vi "Configure_Interrupt_Duration.vi"(7 "I2C Channel":u8, 8 "error in":errorcluster, 9 "Interrupt Threshold":u8, 10 "Interrupt Source":T1(ring), 11 "LINX Resource In":T2) -> (0 "error out":errorcluster, 2 "ODR-adjusted Duration (s)":dbl, 3 "LINX Resource Out":T2)   [LabVIEW 2014, in "LMH-LINX.lvlib" / "LIS331HH.lvlib"]
uses:
  <vilib>/MakerHub/LINX/Public/Sensors/Accelerometer/LIS331HH/LIS331HH.lvlib
  <vilib>/MakerHub/LINX/Private/Type Defs/LINX Ref.ctl
  <vilib>/MakerHub/LINX/Private/Type Defs/Platform.ctl
  <vilib>/MakerHub/LINX/Private/Type Defs/Interface.ctl
  <vilib>/MakerHub/LINX/Private/Device/Type Defs/LINX Device Config.ctl
  <vilib>/MakerHub/LINX/Private/Device/Type Defs/TCP Config.ctl
  <vilib>/MakerHub/LINX/Private/Device/Type Defs/Channels.ctl
  <vilib>/MakerHub/LINX/Private/Local IO/LinxI2cWrite.vi
  <vilib>/MakerHub/LINX/Public/Utilities/Check Channel.vi
  <vilib>/MakerHub/LINX/Private/Utilties/Generate Error.vi
  <vilib>/MakerHub/LINX/LMH-LINX.lvlib
  <vilib>/MakerHub/LINX/Private/Device/Device.lvlib
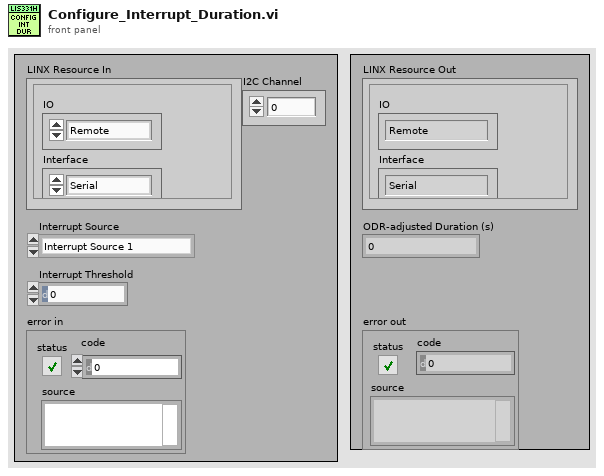
[diagram p1: front panel]
types:
  T1 = enum16{"Interrupt Source 1", "Interrupt Source 2"}
  T2 = typedef "LMH-LINX.lvlib/LINX Ref.ctl" = cluster{"IO":T3, "Interface":T4, "LINX Device Config":T5}
  T3 = typedef "LMH-LINX.lvlib/Platform.ctl" = enum16{"Remote", "Local"}
  T4 = typedef "LMH-LINX.lvlib/Interface.ctl" = enum16{"Serial", "TCP"}
  T5 = typedef "LMH-LINX.lvlib/Device.lvlib/LINX Device Config.ctl" = cluster{"Interface":T4, "COM Port":refnum<visa-resource-name>, "TCP Configuration":T6, "Device Family":u8, "Device ID":u8, "Device Name":string, "TCP Ref":refnum<k5>, "Channels":T7}
  T6 = typedef "LMH-LINX.lvlib/Device.lvlib/TCP Config.ctl" = cluster{"IP Address":string, "Port":u16}
  T7 = typedef "LMH-LINX.lvlib/Channels.ctl" = cluster{"DI":u8[], "DO":u8[], "AI":u8[], "AO":u8[], "PWM":u8[], "QE":u8[], "UART":u8[], "I2C 2":u8[], "SPI":u8[], "CAN":u8[], "Servo":u8[], "AI Ref (V)":dbl, "AI Resolution (Bits)":u8, "AO Ref (V)":dbl, "AO Resolution (Bits)":u8}
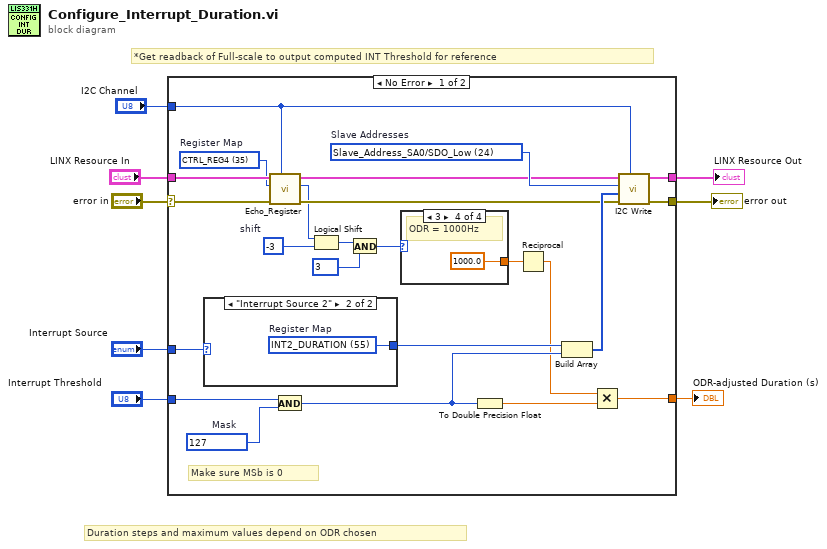
[diagram p0: block diagram]
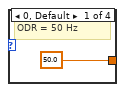
[diagram p2: hidden frame]
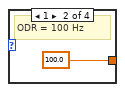
[diagram p3: hidden frame]
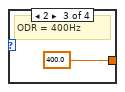
[diagram p4: hidden frame]
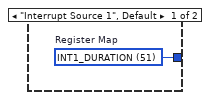
[diagram p5: hidden frame]
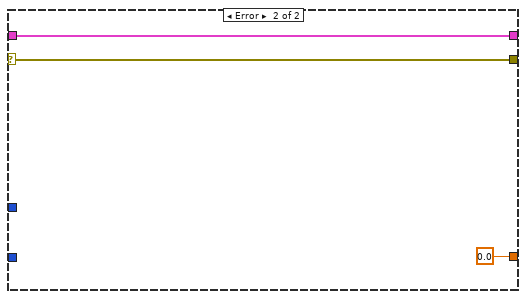
[diagram p6: hidden frame]
diagram:
  # "*Get readback of Full-scale to output computed INT Threshold for reference"
  # "Duration steps and maximum values depend on ODR chosen"
  n1 = case shown="No Error" "error in" {
    selector: "error in" -> [w23 w41]
    tunnel: [w31 w41] -> w7
    tunnel: "LINX Resource In" -> [w24 w40]
    tunnel: "I2C Channel" -> [w20 _]
    tunnel: [w32 w40] -> w4
    tunnel: "Interrupt Source" -> [w29 _]
    tunnel: "Interrupt Threshold" -> [w26 _]
    tunnel: [w14 0.0] -> w1
    frame No Error {
      w17 = i8 -3  # shift
      w19 = u8 35 items=["CTRL_REG1"=32, "CTRL_REG2"=33, "CTRL_REG3"=34, "CTRL_REG4"=35, "CTRL_REG5"=36, "HP_FILTER_RESET"=37, "REFERENCE"=38, "STATUS_REG"=39, "OUT_X_L"=40, "OUT_X_H"=41, "OUT_Y_L"=42, "OUT_Y_H"=43, "OUT_Z_L"=44, "OUT_Z_H"=45, "INT1_CFG"=48, "INT1_SOURCE"=49, "INT1_THS"=50, "INT1_DURATION"=51, "INT2_CFG"=52, "INT2_SOURCE"=53, "INT2_THS"=54, "INT2_DURATION"=55]  # Register Map
      w25 = u8 127  # Mask
      w30 = u8 24 items=["Slave_Address_SA0/SDO_Low"=24, "Slave_Address_SA0/SDO_High"=25]  # Slave Addresses
      # "Make sure MSb is 0"
      n2 = case shown="\"Interrupt Source 2\"" w29 {
        tunnel: [w37 w38] -> w28
        frame "Interrupt Source 1", Default {
          w37 = u8 51 items=["CTRL_REG1"=32, "CTRL_REG2"=33, "CTRL_REG3"=34, "CTRL_REG4"=35, "CTRL_REG5"=36, "HP_FILTER_RESET"=37, "REFERENCE"=38, "STATUS_REG"=39, "OUT_X_L"=40, "OUT_X_H"=41, "OUT_Y_L"=42, "OUT_Y_H"=43, "OUT_Z_L"=44, "OUT_Z_H"=45, "INT1_CFG"=48, "INT1_SOURCE"=49, "INT1_THS"=50, "INT1_DURATION"=51, "INT2_CFG"=52, "INT2_SOURCE"=53, "INT2_THS"=54, "INT2_DURATION"=55]  # Register Map
        }
        frame "Interrupt Source 2" {
          w38 = u8 55 items=["CTRL_REG1"=32, "CTRL_REG2"=33, "CTRL_REG3"=34, "CTRL_REG4"=35, "CTRL_REG5"=36, "HP_FILTER_RESET"=37, "REFERENCE"=38, "STATUS_REG"=39, "OUT_X_L"=40, "OUT_X_H"=41, "OUT_Y_L"=42, "OUT_Y_H"=43, "OUT_Z_L"=44, "OUT_Z_H"=45, "INT1_CFG"=48, "INT1_SOURCE"=49, "INT1_THS"=50, "INT1_DURATION"=51, "INT2_CFG"=52, "INT2_SOURCE"=53, "INT2_THS"=54, "INT2_DURATION"=55]  # Register Map
        }
      }
      n3 = call <vilib>:"Echo_Register.vi"("I2C Channel"=w20, "error in (no error)"=w23, "Register to Echo"=w19, "LINX Resource In"=w24) -> ("error out"=w22:errorcluster, "Register Word"=w18:u8, "LINX Resource Out"=w21:T2)  [unwired: 5 in]
      n4 = And(x=w26, y=w25) -> (x .and. y?=w16:u8)
      n5 = Logical Shift(y=w18, x=w17) -> (x << y=w13:i8)
      n6 = And(x=w13, y=i8 3) -> (x .and. y?=w12:i8)
      n7 = case shown="3" w12 {
        tunnel: [50.0 100.0 400.0 1000.0] -> w10
        frame 0, Default {
          # "ODR = 50 Hz"
        }
        frame 1 {
          # "ODR = 100 Hz"
        }
        frame 2 {
          # "ODR = 400Hz"
        }
        frame 3 {
          # "ODR = 1000Hz"
        }
      }
      n8 = To Double Precision Float(number=w16) -> (double precision float=w15:dbl)
      n9 = Reciprocal(x=w10) -> (1/x=w9:dbl)
      n10 = Build Array(w28, w16) -> (w27:u8[])
      n11 = Multiply(x=w9, y=w15) -> (x*y=w14:dbl)
      n12 = call <vilib>:"I2C Write.vi"("I2C Channel"=w20, "Error In"=w22, "Data"=w27, "I2C Slave Address (0)"=w30, "LINX Resource"=w21) -> ("Error Out"=w31:errorcluster, "LINX Resource"=w32:T2)  [unwired: 5 in]
    }
    frame Error {
    }
  }
  "error out" <- w7
  "LINX Resource Out" <- w4
  "ODR-adjusted Duration (s)" <- w1
